vi "盲元标记.vi"(6 "阈值 2":dbl, 8 "error constant 2":errorcluster, 9 "进度 2":refnum<vi>, 10 "path in":path, 11 "Intensity Graph":dbl[][](graph)) -> (0 "error constant":errorcluster, 1 "盲元表":dbl[][](graph), 2 "盲元标定结果":bool, 3 "盲元总数":dbl)   [LabVIEW 2016]
uses:
  Data/Global.vi
panel:
  out "Numeric":u16
  out "return type 4":i32
  out "return type 3":i32
  out "return type 2":i32
  out "return type":i32
  in  "阈值":dbl=1500.0
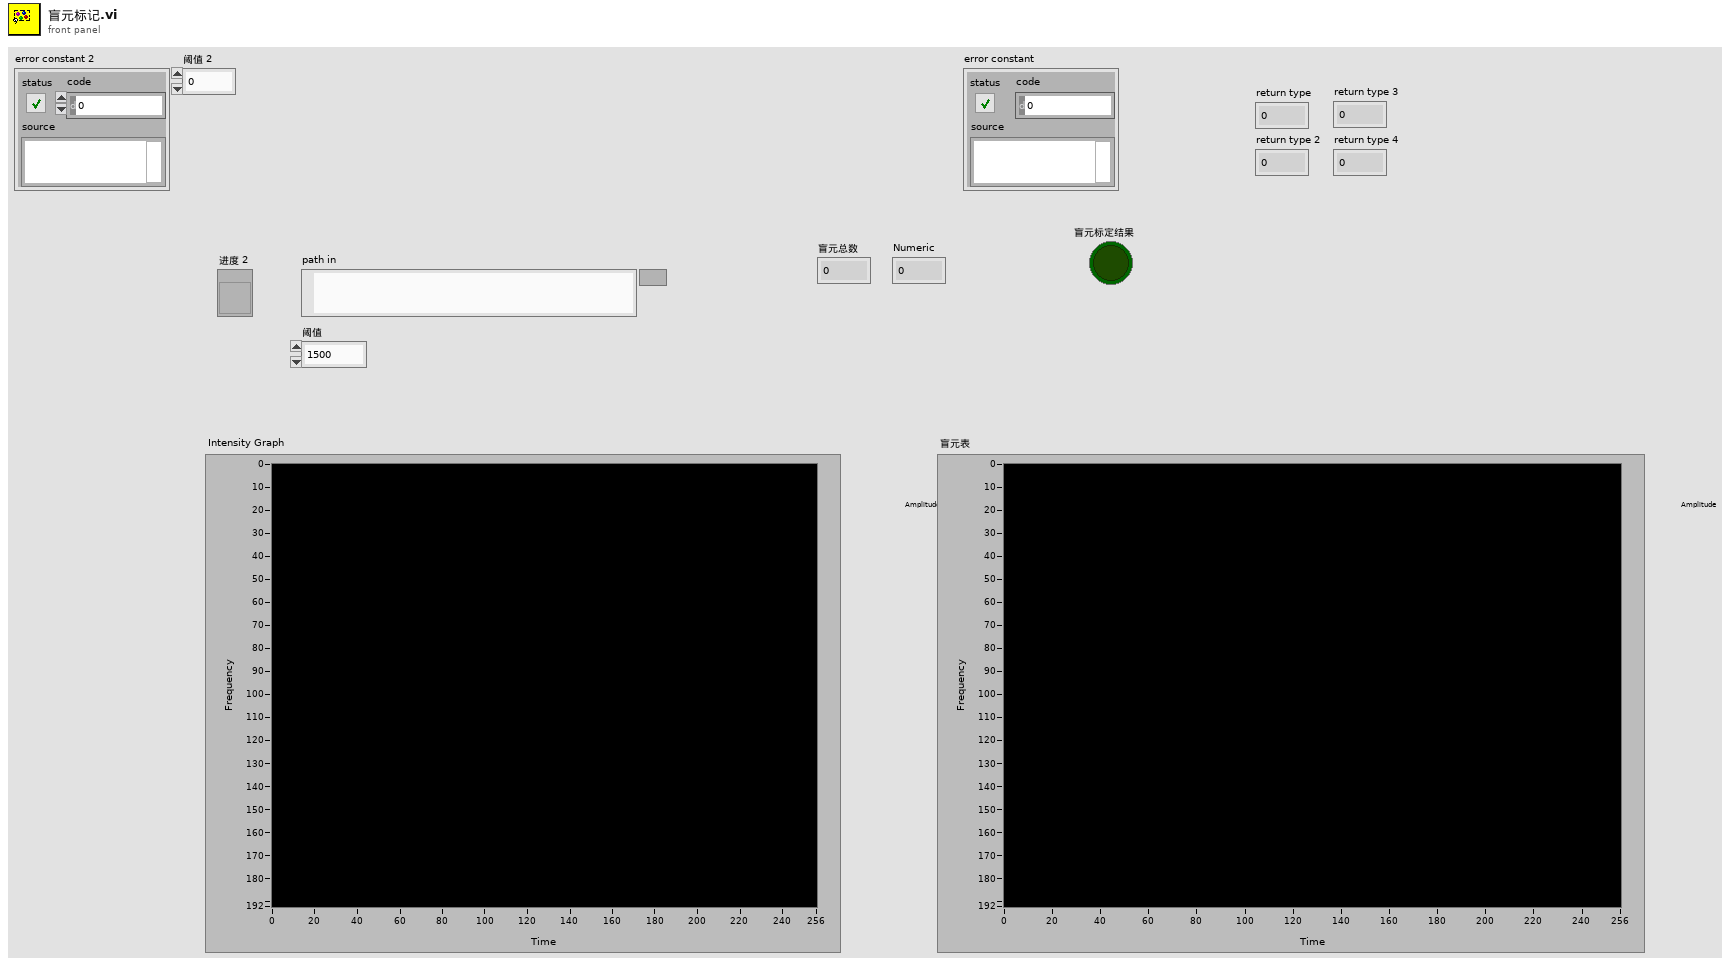
[diagram p1: front panel]
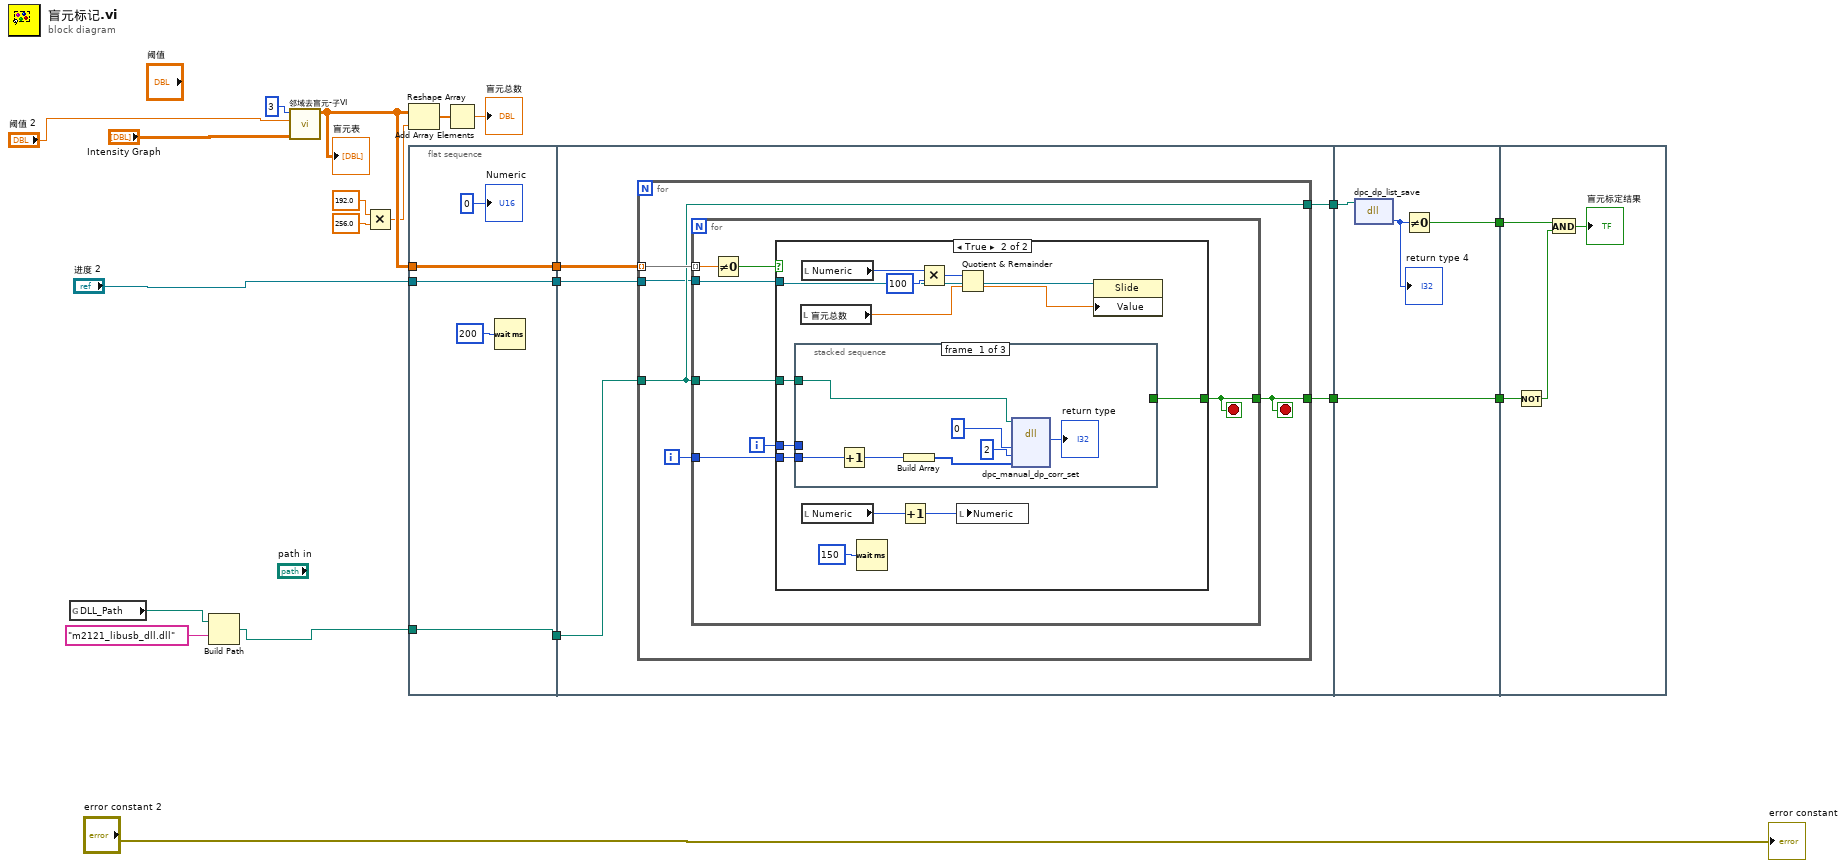
[diagram p0: block diagram]
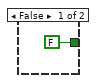
[diagram p2: hidden frame]
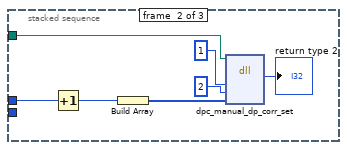
[diagram p3: hidden frame]
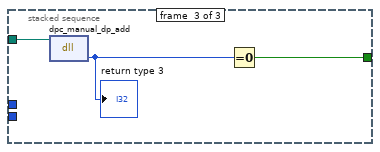
[diagram p4: hidden frame]
diagram:
  n1 = global read "Global.vi" "DLL_Path"() -> (w8:path)
  n2 = Build Path(base path=w8, name or relative path="m2121_libusb_dll.dll") -> (appended path=w6:path)
  n3 = call "邻域去盲元-子VI.vi"("输入"="Intensity Graph", "阈值"="阈值 2", "尺寸"=3) -> ("盲元表"=w18:dbl[][])  [unwired: 7 in, 1 out]
  "盲元表" <- w18
  n4 = Multiply(x=192.0, y=256.0 ("x")) -> (x*y=w15:dbl)
  n5 = Reshape Array(w18, w15) -> (w14:dbl[])
  n6 = flat-sequence {
    tunnel: [w26] -> w10
    tunnel: w6 -> [w22]
    tunnel: w18 -> [w26]
    tunnel: "进度 2" -> [w23]
    tunnel: [w23] -> w5
    tunnel: [w22] -> w2
    tunnel: [w30] -> w19
    tunnel: [w29] -> w12
    tunnel: w10 -> [w31]
    tunnel: w5 -> [w28]
    tunnel: w2 -> [w27]
    tunnel: w19 -> [w78]
    tunnel: [w77] -> w13
    tunnel: w12 -> [w77]
    tunnel: [w75] -> w11
    tunnel: w13 -> [w82]
    tunnel: w11 -> [w81]
    frame #0 {
      n7 = Wait (ms)(milliseconds to wait=u32 200) -> ()  [unwired: 1 out]
      "Numeric" <- 0
    }
    frame #1 {
      n8 = for {
        tunnel: w31 -> [w36] mode=indexing
        tunnel: w27 -> [w35]
        tunnel: [w35] -> w30
        tunnel: [w33] -> w29
        tunnel: w28 -> [w32]
        i -> [w34]
        stop <- w33 stop-if-true
        n9 = for {
          tunnel: w36 -> [w43] mode=indexing
          tunnel: w34 -> [w41]
          tunnel: w35 -> [w39]
          tunnel: [w38] -> w33
          tunnel: w32 -> [w37]
          i -> [w40]
          stop <- w38 stop-if-true
          n10 = Not Equal To 0?(x=w43) -> (x != 0?=w42:bool)
          n11 = case shown="True" w42 {
            tunnel: w41 -> [_ w57]
            tunnel: w40 -> [_ w56]
            tunnel: w39 -> [_ w55]
            tunnel: [FALSE w53] -> w38
            tunnel: w37 -> [_ w46]
            frame False {
            }
            frame True {
              n12 = stacked-sequence {
                tunnel: w57 -> [w61 _ _]
                tunnel: w55 -> [w59 w66 w74]
                tunnel: w56 -> [_ w68 _]
                tunnel: [_ _ w72] -> w53
                frame #0 {
                  n13 = Increment(x=w61) -> (x+1=w60:i32)
                  n14 = Build Array(w60) -> (w62:i32[])
                  n15 = dll-call lib="PTH24abs J小模组调试datam2121_libusb_dll.dll" fn="dpc_manual_dp_corr_set"(path in=w59, "arg1"=0, "arg2"=2 ("arg1"), "arg3"=w62) -> ("return type"=→"return type":i32)  [unwired: 5 in, 2 out]
                }
                frame #1 {
                  n16 = Increment(x=w68) -> (x+1=w67:i32)
                  n17 = Build Array(w67) -> (w71:i32[])
                  n18 = dll-call lib="PTH24abs J小模组调试datam2121_libusb_dll.dll" fn="dpc_manual_dp_corr_set"(path in=w66, "arg1"=1, "arg2"=2 ("arg1"), "arg3"=w71) -> ("return type"=→"return type 2":i32)  [unwired: 5 in, 2 out]
                }
                frame #2 {
                  n19 = dll-call lib="PTH2Kabs F工作\nlabview程序小模组调试datam2121_libusb_dll.dll" fn="dpc_manual_dp_add"(path in=w74) -> ("return type"=w73:i32)  [unwired: 2 in, 2 out]
                  "return type 3" <- w73
                  n20 = Equal To 0?(x=w73) -> (x = 0?=w72:bool)
                }
              }
              n21 = local read "盲元总数"() -> (w50:dbl)
              n22 = local read "Numeric"() -> (w48:u16)
              n23 = local read "Numeric"() -> (w52:u16)
              n24 = Wait (ms)(milliseconds to wait=u32 150) -> ()  [unwired: 1 out]
              n25 = Increment(x=w52) -> (x+1=w51:u16)
              n26 = Multiply(x=w48, y=100) -> (x*y=w47:i32)
              n27 = local write "Numeric"(w51) -> ()
              n28 = Quotient & Remainder(x=w47, y=w50) -> (floor(x/y)=w45:dbl)  [unwired: 1 out]
              n29 = property class="Slide"(reference=w46, "Value"=w45) -> ()  [unwired: 1 in, 2 out]
            }
          }
        }
      }
    }
    frame #2 {
      n30 = dll-call lib="PTH2Kabs F工作\nlabview程序小模组调试datam2121_libusb_dll.dll" fn="dpc_dp_list_save"(path in=w78) -> ("return type"=w76:i32)  [unwired: 2 in, 2 out]
      "return type 4" <- w76
      n31 = Not Equal To 0?(x=w76) -> (x != 0?=w75:bool)
    }
    frame #3 {
      n32 = Not(x=w82) -> (.not. x?=w80:bool)
      n33 = And(x=w81, y=w80) -> (x .and. y?=→"盲元标定结果":bool)
    }
  }
  n34 = Add Array Elements(numeric array=w14) -> (sum=→"盲元总数":dbl)
  "error constant" <- "error constant 2"
